vi "Connect.vi"(8 "error in":errorcluster, 11 "89XX in":refnum<class "89XX.lvclass">) -> (0 "error out":errorcluster, 3 "89XX out":refnum<class "89XX.lvclass">)   [LabVIEW 2019, in "89XX.lvlib" / "89XX.lvclass"]
uses:
  Library/89XX.lvclass
  C:/Users/Public/Documents/Development/builds/Instruments/Instruments.lvlibp/Library/Instruments.lvclass
  Library/89XX.lvclass/89XX.ctl
  builds/Instruments/Instruments.lvlibp/Accessors/Read Resource.vi
  <instrlib>/Keysight N8900 Series/Keysight N8900 Series.lvlib
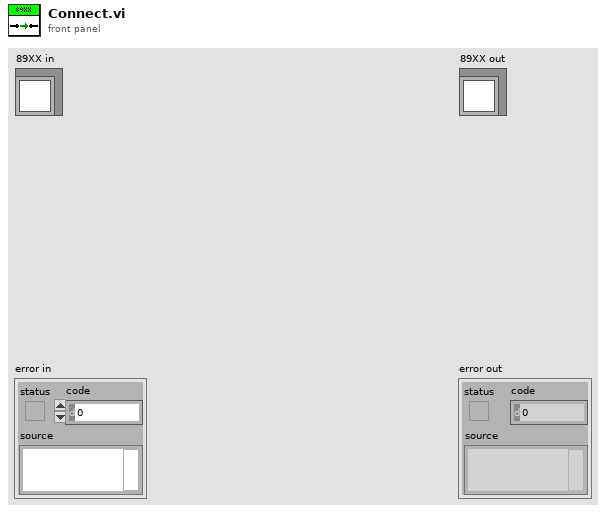
[diagram p1: front panel]
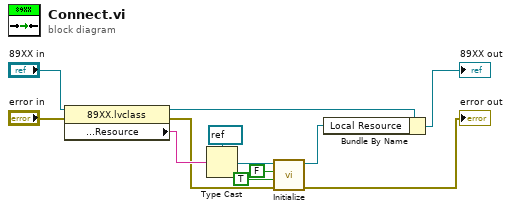
[diagram p0: block diagram]
diagram:
  n1 = property class="89XX.lvclass"(reference="89XX in", error in="error in") -> (reference out=w4:refnum<class "89XX.lvclass">, error out=w7:errorcluster, "Accessors:Configuration:Resource"=w10:string)
  n2 = Type Cast(type=refnum<visa-resource-name> refnum ("VISA resource name"), x=w10) -> (*(type *) &x=w8:refnum<visa-resource-name>)
  n3 = call <instrlib>:"Initialize.vi"("error in (no error)"=w7, "Reset (True)"=TRUE, "ID Query (True)"=FALSE, "VISA resource name"=w8) -> ("error out"=→"error out":errorcluster, "VISA resource name out"=w3:refnum<visa-resource-name>)  [unwired: 6 in]
  n4 = Bundle By Name(cluster=w4, "Local Resource"=w3) -> (→"89XX out":refnum<class "89XX.lvclass">)
